vi "Destroy Message-Enqueuer References.vi"(8 "error in (no error)":errorcluster, 11 "Event-References":T1) -> (0 "error out":errorcluster)   [LabVIEW 2018, in "Scripting.lvlib" / "Actor.lvclass"]
uses:
  Actor.lvclass
  All-Enqueuers.ctl
  Broadcast Enqueuers.ctl
  Did Initialize.ctl
  Request-Enqueuers.ctl
  Get State.ctl
  State.ctl
  Stop.ctl
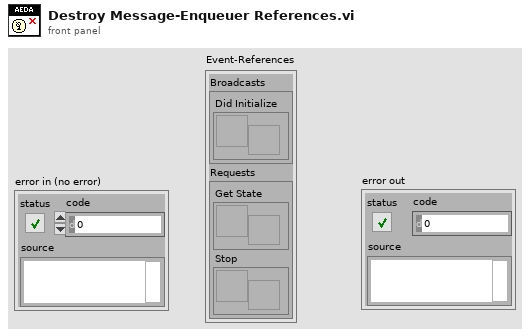
[diagram p1: front panel]
types:
  T1 = typedef "Scripting.lvlib/Actor.lvclass/All-Enqueuers.ctl" = cluster{"Broadcasts":T2, "Requests":T3}
  T2 = typedef "Scripting.lvlib/Actor.lvclass/Broadcast Enqueuers.ctl" = cluster{"Did Initialize":refnum<user-event>}
  T3 = typedef "Scripting.lvlib/Actor.lvclass/Request-Enqueuers.ctl" = cluster{"Get State":refnum<user-event>, "Stop":refnum<user-event>}
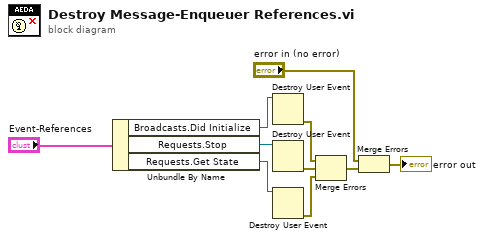
[diagram p0: block diagram]
diagram:
  n1 = Unbundle By Name("Event-References") -> ("Broadcasts.Did Initialize"=w9:refnum<user-event>, "Requests.Stop"=w8:refnum<user-event>, "Requests.Get State"=w7:refnum<user-event>)
  n2 = Destroy User Event(user event=w9) -> (error out=w6:errorcluster)  [unwired: 1 in]
  n3 = Destroy User Event(user event=w8) -> (error out=w5:errorcluster)  [unwired: 1 in]
  n4 = Destroy User Event(user event=w7) -> (error out=w4:errorcluster)  [unwired: 1 in]
  n5 = Merge Errors(w6, w5, w4) -> (w1:errorcluster)
  n6 = Merge Errors("error in (no error)", w1) -> (→"error out":errorcluster)
